vi "Echo Parameters.vi"   [LabVIEW 2017, in "Integration Tests.lvlib"]
uses:
  Integration Tests.lvlib
  CLI Class/CLI.lvclass
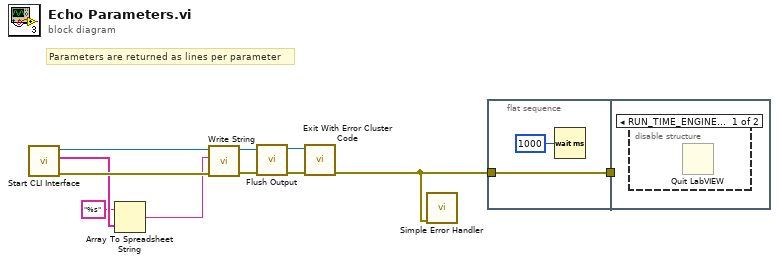
[diagram p0: block diagram]
diagram:
  # "Parameters are returned as lines per parameter"
  n1 = call "Start CLI Interface.vi"() -> ("error out"=w9:errorcluster, "Custom Parameters"=w8:string[], "CLI out"=w10:refnum<class "CLI.lvclass">)  [unwired: 8 in, 1 out]
  n2 = Array To Spreadsheet String(array=w8, 3:"%s" ("format string")) -> (spreadsheet string=w6:string)  [unwired: 1 in]
  n3 = call "Write String.vi"("error in (no error)"=w9, "Text to Write"=w6, "CLI in"=w10) -> ("error out"=w11:errorcluster, "CLI out"=w2:refnum<class "CLI.lvclass">)  [unwired: 7 in]
  n4 = call "Flush Output.vi"("error in (no error)"=w11, "CLI in"=w2) -> ("error out"=w3:errorcluster, "CLI out"=w1:refnum<class "CLI.lvclass">)  [unwired: 8 in]
  n5 = call "Exit With Error Cluster Code.vi"("error in (no error)"=w3, "CLI in"=w1) -> ("error out"=w4:errorcluster)  [unwired: 9 in]
  n6 = call <vilib>:"Simple Error Handler.vi"("error in (no error)"=w4) -> ()  [unwired: 4 in, 5 out]
  n7 = flat-sequence {
    tunnel: w4 -> [w13]
    tunnel: [w13] -> w5
    tunnel: w5 -> [_]
    frame #0 {
      n8 = Wait (ms)(milliseconds to wait=u32 1000) -> ()  [unwired: 1 out]
    }
    frame #1 {
      n9 = disable-structure shown="RUN_TIME_ENGINE==True" {
        frame condition #0 {
          n10 = Quit LabVIEW() -> ()  [unwired: 1 in]
        }
        frame condition #1 (active) {
        }
      }
    }
  }
